vi "lab #4.vi"(9 "C":dbl, 10 "B":dbl, 11 "A":dbl) -> (2 "Area":dbl, 3 "S":dbl)   [LabVIEW 2016]
panel:
  out "Valid Triangle":bool
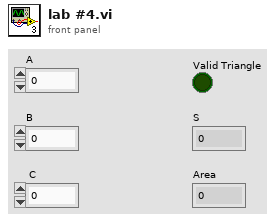
[diagram p1: front panel]
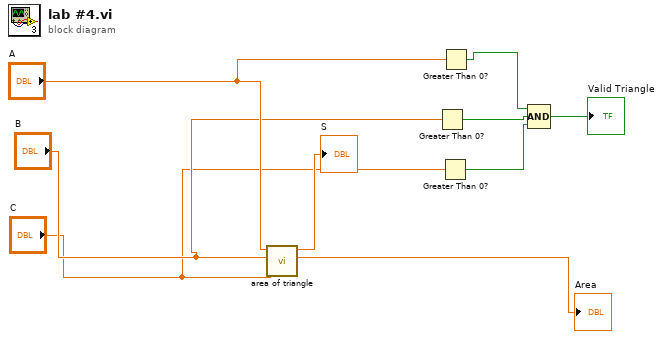
[diagram p0: block diagram]
diagram:
  n1 = call "area of triangle.vi"("C"="C", "B"="B", "A"="A") -> ("Area"=→"Area":dbl, "S"=→"S":dbl)  [unwired: 7 in]
  n2 = Greater Than 0?(x="B") -> (x > 0?=w6:bool)
  n3 = Greater Than 0?(x="C") -> (x > 0?=w5:bool)
  n4 = Greater Than 0?(x="A") -> (x > 0?=w7:bool)
  n5 = Compound Arithmetic op=AND(w7, w6, w5) -> (→"Valid Triangle":bool)
